vi "AMmoddemodtest.vi"() -> ()   [LabVIEW 2011]
panel:
  out "Rx Signal":dbl[](array[numeric])
  in  "Fs":dbl
  in  "Fc":dbl
  in  "Tx Signal":dbl[](array[numeric])
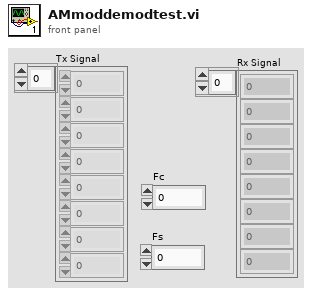
[diagram p1: front panel]
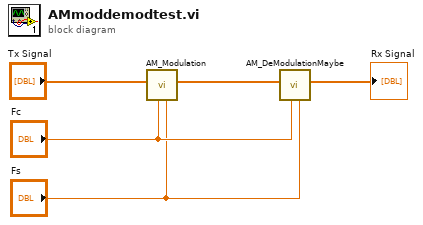
[diagram p0: block diagram]
diagram:
  n1 = call "AM_Modulation.vi"("Fs"="Fs", "Fc"="Fc", "message"="Tx Signal") -> ("mod_signal"=w2:dbl[])  [unwired: 8 in]
  n2 = call "AM_DeModulationMaybe.vi"("Fs"="Fs", "Fc"="Fc", "mod_signal"=w2) -> ("message"=→"Rx Signal":dbl[])  [unwired: 8 in]
